vi "PCO_SetCameraRamSegmentSize.vi"(8 "error in (no error)":errorcluster {"code" format="%x"}, 10 "dwRamSegSize":u32[](array[numeric])=[0, 0, 0, 0], 11 "ph":u64) -> (0 "error out":errorcluster {"code" format="%x"}, 2 "ErrorMessage":i32 format="%x", 3 "ph out":u64)   [LabVIEW 2019, in "SDK.lvlib" / "StorageControl.lvlib"]
doc: "<b>Description:</b>\nThis function does set segment size in CamRAM pages of the four memory segments. The segment size must be large enough to hold at least two images. All image data in all segments is cleared.\n\n<b>All previously recorded images will be lost.</b>\n• The sum of all segment sizes must not be larger than the total size of the RAM \n (as multiples of pages).\n• A single segment size can have the value 0x0000, but the sum of all four segments must be \n bigger than the size of two images.\n• Pay attention that the array dwRamSegSize is zero based indexed while the segment number \n is 1 based, e.g. RAM size of segment 1 is stored in dwRamSegSize[0].\n• The command will be rejected, if Recording State is [run], see PCO_GetRecordingState.\n\n<b>Supported camera type:</b>\npco.dimax, pco.1200, pco.1600, pco.2000, pco.4000\n\n<b>Descriptor dependency:</b>\ndwGeneralCapsDESC1: NO_RECORDER"
uses:
  StorageControl.lvlib
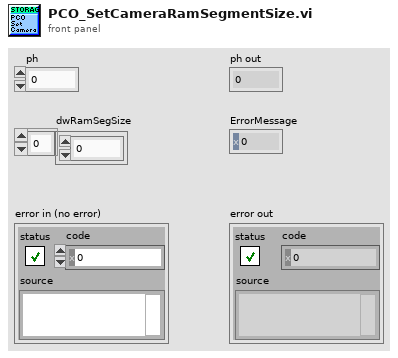
[diagram p1: front panel]
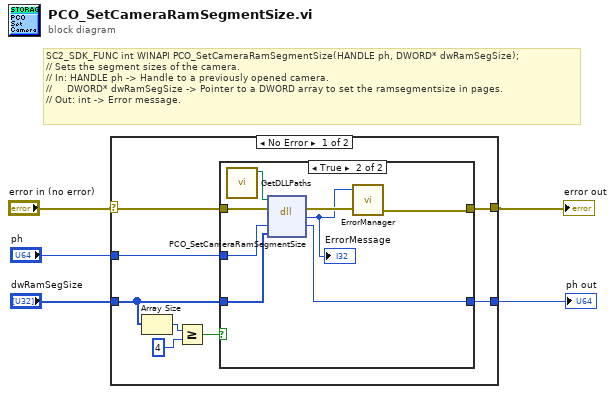
[diagram p0: block diagram]
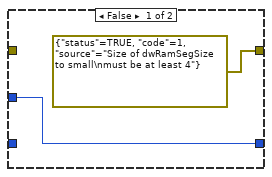
[diagram p2: hidden frame]
diagram:
  # "SC2_SDK_FUNC int WINAPI PCO_SetCameraRamSegmentSize(HANDLE ph, DWORD* dwRamSegSize);\n// Sets the segment sizes of the camera.\n// In: HANDLE ph -> Handle to a previously opened camera.\n//     DWORD* dwRamSegSize -> Pointer to a DWORD array to set the ramsegmentsize in pages.\n// Out: int -> Error message."
  n1 = case shown="No Error" "error in (no error)" {
    selector: "error in (no error)" -> [w11 w25]
    tunnel: "ph" -> [w13 w24]
    tunnel: [w12 w24] -> w4
    tunnel: "dwRamSegSize" -> [w10 _]
    tunnel: [w6 w25] -> w1
    frame No Error {
      n2 = Array Size(array=w10) -> (size(s)=w9:i32)
      n3 = Greater Or Equal?(x=w9, y=4) -> (x >= y?=w7:bool)
      n4 = case shown="True" w7 {
        tunnel: w13 -> [w15 w23]
        tunnel: [w15 w22] -> w12
        tunnel: [errorcluster {"status"=TRUE, "code"=1, "source"="Size of dwRamSegSize to small\nmust be at least 4"} ("error out") w18] -> w6
        tunnel: w11 -> [_ w21]
        tunnel: w10 -> [_ w20]
        frame False {
        }
        frame True {
          n5 = call "GetDLLPaths.vi"() -> ("SC2_Cam_Path"=w16:path)  [unwired: 8 in, 3 out]
          n6 = dll-call lib="?" fn="PCO_SetCameraRamSegmentSize"(path in=w16, error in=w21, "ph"=w23, "dwRamSegSize"=w20) -> (error out=w19:errorcluster, "return type"=w17:i32, "ph"=w22:u64)  [unwired: 2 in, 1 out]
          "ErrorMessage" <- w17
          n7 = call "ErrorManager.vi"("error in (no error)"=w19, "error code"=w17) -> ("error out"=w18:errorcluster)  [unwired: 2 in, 1 out]
        }
      }
    }
    frame Error {
    }
  }
  "ph out" <- w4
  "error out" <- w1
